vi "desaccade operation.vi"(0 "Data not diff":dbl[][](array[numeric]), 7 "Parameter":T1={"Threshold 1 [Acc]"=0.0, "Threshold 2 [% of TH1]"=0, "tolerance"=2.0, "Search WD "=0.05757575757575758, " always use TH2"=TRUE, "SD for Outliers"=3.0303030303030303, "Max time [ms]"=50.0, "Min time [ms]"=1.0, "Velocity Threshold"=0.05757575757575758} {"Velocity Threshold" scale=50.0..400.0; "SD for Outliers" scale=0.0..5.0; "Search WD" scale=0.0..0.3; "tolerance" scale=0.0..100.0; "Threshold 2 [% of TH1]" scale=0.0..100.0; "Threshold 1 [Acc]" scale=1.0..40000.0}, 11 "Sample Rate":dbl=500.0 format="%.2f") -> (4 "Desaccaded":dbl[][](graph))   [LabVIEW 2016, in "Desaccade Manipulator.lvclass"]
uses:
  Desaccade Manipulator.lvclass
  Typedef - Desaccading Parameter.ctl
  <vilib>/Analysis/3filter.llb/Savitzky-Golay Filter (DBL).vi
  <vilib>/Analysis/NI_AALPro.lvlib
  <vilib>/Analysis/NI_AALBase.lvlib
  comm/nan operations/nan operations.lvlib
panel:
  out "Desaccaded 4":dbl[](graph)
  out "Saccades":dbl[][](graph)
  out "Data Diff & Quadr - Unsmoothed":dbl[][](graph)
  out "Data DIff & Quadr - Smoothed":dbl[][](graph)
  out "Data not differentiated":dbl[][](graph)
  # "Data Input"
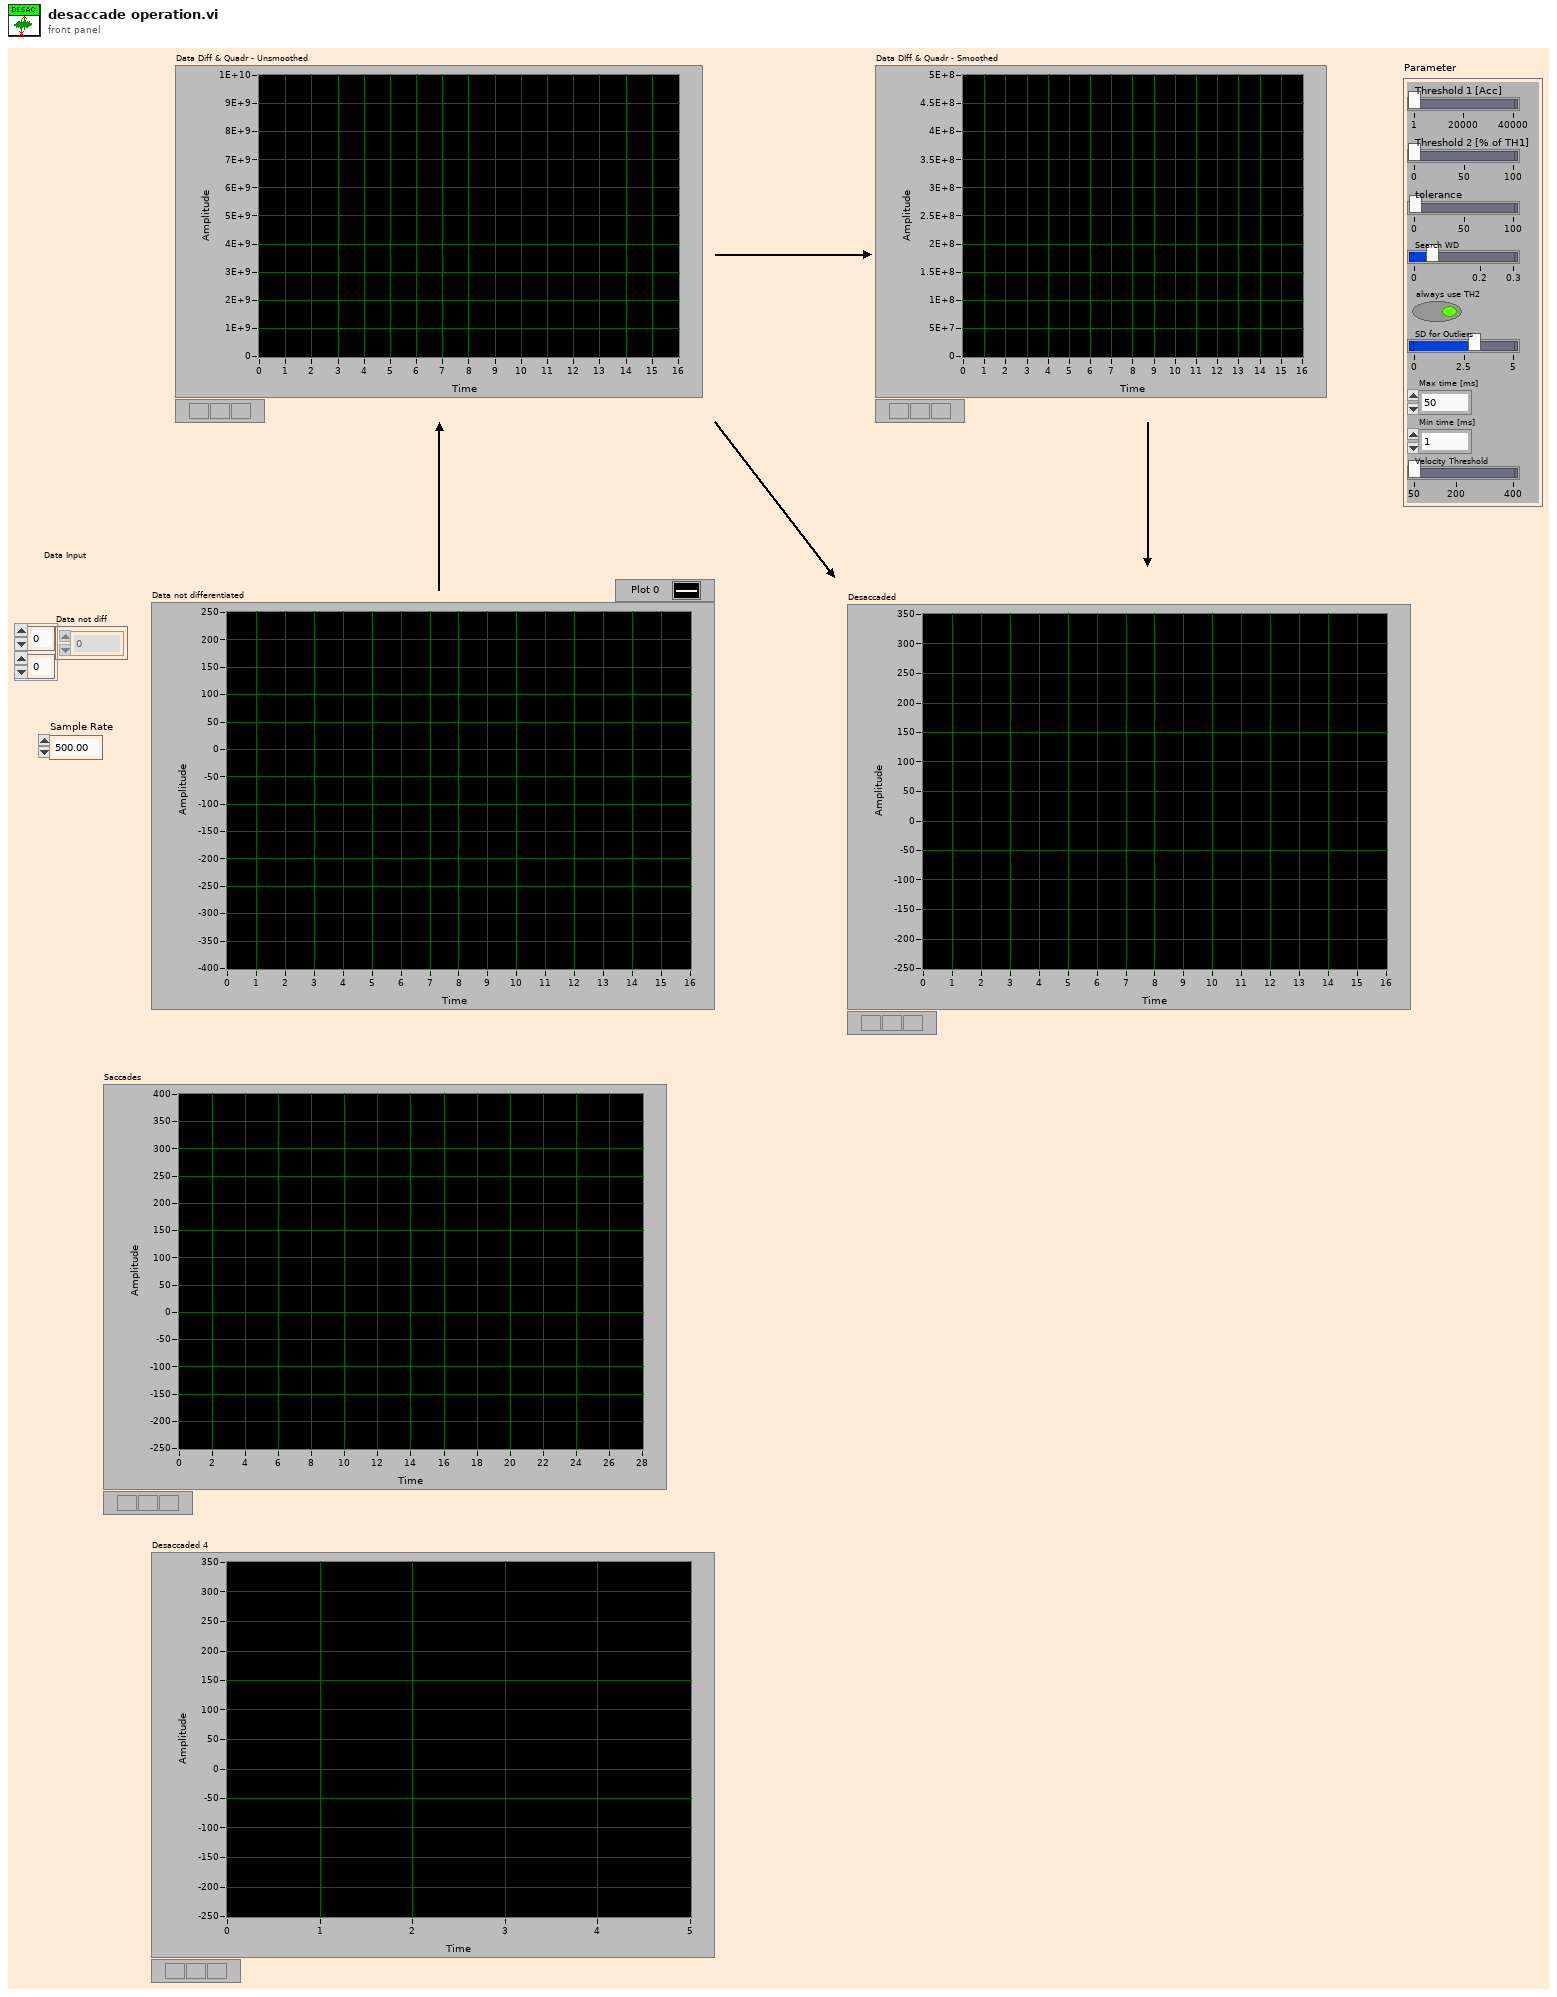
[diagram p1: front panel]
types:
  T1 = typedef "Typedef - Desaccading Parameter.ctl" = cluster{"Threshold 1 [Acc]":dbl, "Threshold 2 [% of TH1]":i32, "tolerance":dbl, "Search WD ":dbl, " always use TH2":bool, "SD for Outliers":dbl, "Max time [ms]":dbl, "Min time [ms]":dbl, "Velocity Threshold":dbl}
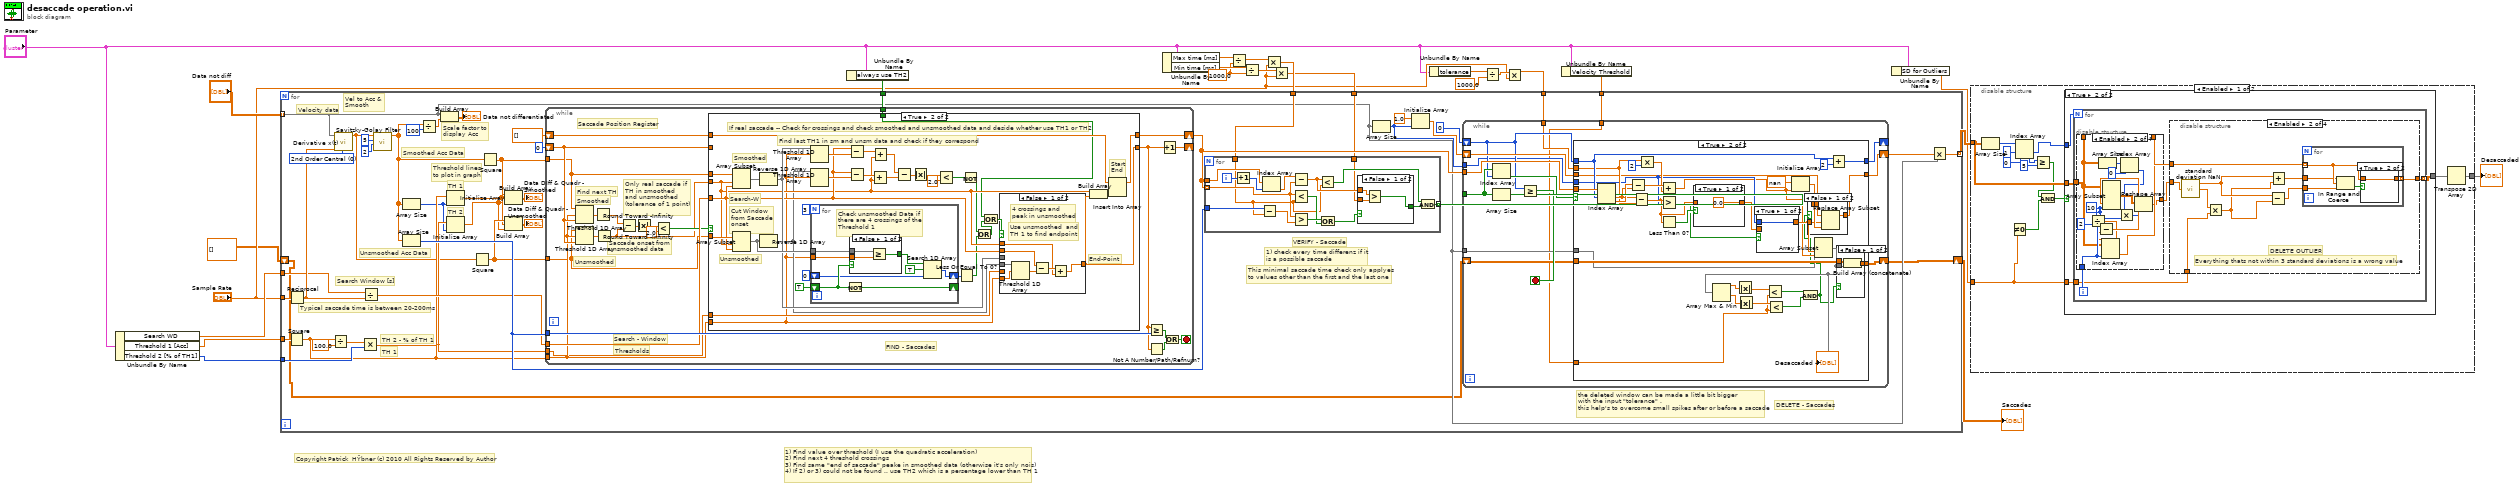
[diagram p0: block diagram]
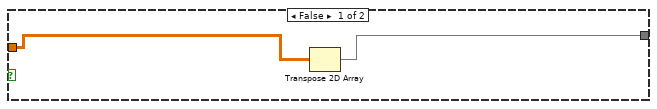
[diagram p2: hidden frame]
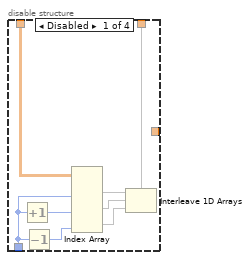
[diagram p3: hidden frame]
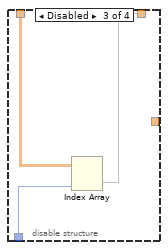
[diagram p4: hidden frame]
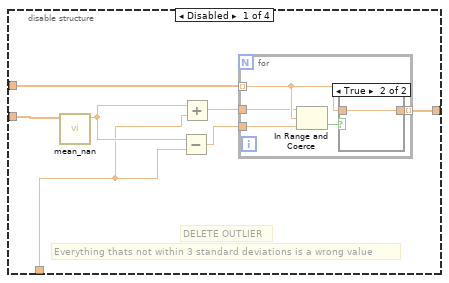
[diagram p6: hidden frame]
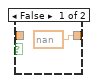
[diagram p7: hidden frame]
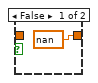
[diagram p8: hidden frame]
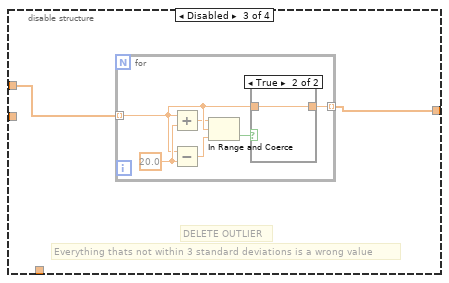
[diagram p9: hidden frame]
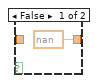
[diagram p10: hidden frame]
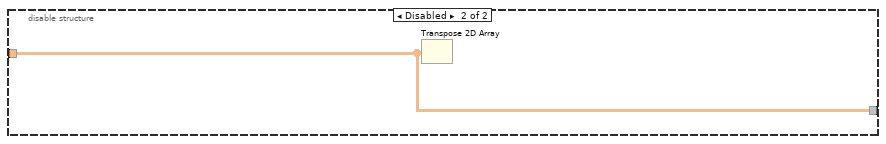
[diagram p12: hidden frame]
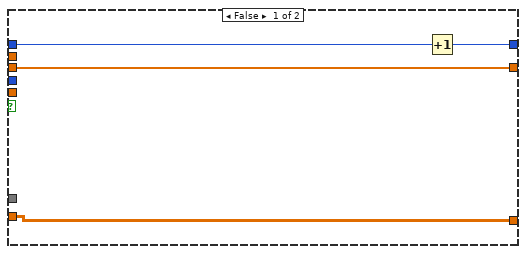
[diagram p13: hidden frame]
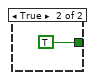
[diagram p18: hidden frame]
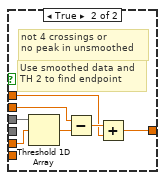
[diagram p20: hidden frame]
diagram:
  w15 = 1000.0 ("y")
  # "1) Find value over threshold (I use the quadratic acceleration)\n2) Find next 4 threshold crossings\n3) Find same \"end of saccade\" peake in smoothed data (otherwise it's only nois)\n4) If 2) or 3) could not be found .. use TH2 which is a persentage lower than TH 1"
  # "Copyright Patrick  HŸbner (c) 2010 All Rights Reserved by Author"
  n1 = Unbundle By Name("Parameter") -> ("Search WD"=w22:dbl, "Threshold 1 [Acc]"=w21:dbl, "Threshold 2 [% of TH1]"=w20:i32)
  n2 = Unbundle By Name("Parameter") -> ("always use TH2"=w19:bool)
  n3 = Unbundle By Name("Parameter") -> ("Max time [ms]"=w17:dbl, "Min time [ms]"=w16:dbl)
  n4 = Divide(x=w17, y=w15) -> (x/y=w14:dbl)
  n5 = Divide(x=w16, y=w15) -> (x/y=w13:dbl)
  n6 = Multiply(x=w14, y="Sample Rate") -> (x*y=w12:dbl)
  n7 = Multiply(x=w13, y="Sample Rate") -> (x*y=w11:dbl)
  n8 = Unbundle By Name("Parameter") -> ("tolerance"=w10:dbl)
  n9 = Divide(x=w10, y=1000.0) -> (x/y=w7:dbl)
  n10 = Multiply(x=w7, y="Sample Rate") -> (x*y=w8:dbl)
  n11 = Unbundle By Name("Parameter") -> ("Velocity Threshold"=w1:dbl)
  n12 = for {
    tunnel: "Sample Rate" -> [w68]
    tunnel: w21 -> [w65]
    tunnel: "Data not diff" -> [w29] mode=indexing
    tunnel: [w35] -> w23 mode=indexing
    tunnel: w20 -> [w51]
    tunnel: w22 -> [w34]
    tunnel: w19 -> [w33]
    tunnel: w12 -> [w32]
    tunnel: w8 -> [w31]
    tunnel: w11 -> [w30]
    shift-right: [w28] -> w3
    shift-left: dbl[][] [] -> [w27]
    tunnel: w1 -> [w26]
    w67 = u16 0 items=["2nd Order Central", "4th Order Central", "Forward", "Backward"] ("method")
    # "DELETE - Saccades"
    # "Scale factor to \ndisplay Acc"
    # "This minimal saccade time check only applyes \nto values other than the first and the last one"
    # "VERIFY - Saccade"
    # "Threshold lines \nto plot in graph"
    # "TH 2"
    # "TH 1"
    # "Vel to Acc &\nSmooth"
    # "Unsmoothed Acc Data"
    # "Smoothed Acc Data"
    # "Velocity data"
    # "Typical saccade time is between 20-200ms"
    # "Search Window [s]"
    # "TH 1"
    # "TH 2 - % of TH 1"
    # "the deleted window can be made a little bit bigger \nwith the input \"tolerance\" . \nthis help's to overcome small spikes after or before a saccade"
    # "1) check every time differenz if it \nis a possible saccade"
    n13 = Square(x=w65) -> (x^2=w47:dbl)
    n14 = Reciprocal(x=w68) -> (1/x=w38:dbl)
    n15 = Divide(x=w47, y=100.0) -> (x/y=w52:dbl)
    n16 = call <vilib>:"Derivative x(t).vi"("method"=w67, "dt"=w38, "X"=w29) -> ("dX/dt"=w25:dbl[])  [unwired: 7 in, 1 out]
    n17 = Multiply(x=w52, y=w51) -> (x*y=w46:dbl)
    n18 = Divide(x=w34, y=w38) -> (x/y=w48:dbl)
    n19 = call-poly <vilib>:"Savitzky-Golay Filter.vi"("polynomial order"=2, "side points"=5, "X"=w25) -> ("Filtered X"=w37:dbl[])  [unwired: 7 in, 1 out]
    n20 = Array Size(array=w37) -> (size(s)=w45:i32)
    n21 = Array Size(array=w37) -> (size(s)=w58:i32)
    n22 = Divide(x=w37, y=100 ("Numeric")) -> (x/y=w55:dbl[])
    n23 = Build Array(w29, w55) -> (→"Data not differentiated":dbl[][])
    n24 = Initialize Array(w47, w45) -> (w40:dbl[])
    n25 = Initialize Array(w46, w45) -> (w39:dbl[])
    n26 = Square(x=w25) -> (x^2=w42:dbl[])
    n27 = Square(x=w37) -> (x^2=w41:dbl[])
    n28 = Build Array(w41, w40, w39) -> (→"Data DIff & Quadr - Smoothed":dbl[][])
    n29 = Build Array(w42, w40, w39) -> (→"Data Diff & Quadr - Unsmoothed":dbl[][])
    n30 = while {
      tunnel: w41 -> [w160]
      shift-right: [w174] -> _
      shift-left: 0 -> [w163]
      shift-right: [w175] -> w60
      shift-left: dbl[] [] ("Filtered X") -> [w173]
      tunnel: w58 -> [w168]
      tunnel: w42 -> [w159]
      tunnel: w48 -> [w165]
      tunnel: w46 -> [w161]
      tunnel: w47 -> [w162]
      tunnel: w33 -> [w154]
      stop <- w167 stop-if-true
      # "FIND - Saccades"
      # "Saccade Position Register"
      # "Only real saccade if\nTH in smoothed\nand unsmoothed \n(tolerance of 1 point)"
      # "Unsmoothed"
      # "Smoothed"
      # "Saccade onset from\nunsmoothed data"
      # "Search - Window"
      # "Thresholds"
      # "Find next TH"
      n31 = Threshold 1D Array(1:w163, 2:w162, 3:w160) -> (0:w176:dbl)
      n32 = Threshold 1D Array(1:w163, 2:w162, 3:w159) -> (0:w172:dbl)
      n33 = Round Toward -Infinity(1:w176) -> (0:w158:dbl)
      n34 = Round Toward -Infinity(1:w172) -> (0:w157:dbl)
      n35 = Subtract(x=w158, y=w157) -> (x-y=w171:dbl)
      n36 = Absolute Value(x=w171) -> (abs(x)=w170:dbl)
      n37 = Less?(x=w170, y=2.0) -> (x < y?=w164:bool)
      n38 = case shown="True" w164 {
        tunnel: [w177 w211] -> w175
        tunnel: w173 -> [w177 w210]
        tunnel: w159 -> [_ w202]
        tunnel: w160 -> [_ w201]
        tunnel: w161 -> [_ w190]
        tunnel: [w178 w189] -> w166
        tunnel: w165 -> [_ w188]
        tunnel: w157 -> [_ w187]
        tunnel: w162 -> [_ w185]
        tunnel: w163 -> [w178 _]
        tunnel: w154 -> [_ w179]
        frame False {
          # "If no real saccade -- Do nothing"
        }
        frame True {
          # "End-Point"
          # "If real saccade -- Check for crossings and check smoothed and unsmoothed data and deside whether use TH1 or TH2"
          # "Find last TH1 in sm and unsm data and check if they correspond"
          # "Smoothed"
          # "Unsmoothed"
          # "Cut Window \nfrom Saccade\nonset"
          # "Search-W"
          # "Start\nEnd"
          n39 = Array Subset(array=w201, index=w187, length=w188) -> (w200:dbl[])
          n40 = Array Subset(array=w202, index=w187, length=w188) -> (w206:dbl[])
          n41 = Reverse 1D Array(array=w200) -> (reversed array=w191:dbl[])
          n42 = Reverse 1D Array(array=w206) -> (reversed array=w186:dbl[])
          n43 = Threshold 1D Array(2:w185, 3:w191) -> (0:w192:dbl)  [unwired: 1 in]
          n44 = Threshold 1D Array(2:w185, 3:w186) -> (0:w199:dbl)  [unwired: 1 in]
          n45 = for {
            N: 3 -> [_]
            tunnel: w206 -> [w233]
            shift-right: [w228] -> _
            shift-left: TRUE -> [w227]
            tunnel: w185 -> [w232]
            shift-right: [w229] -> w203
            shift-left: 0 ("index of element") -> [w226]
            # "Check unsmoothed Data if \nthere are 4 crossings of the \nThreshold 1"
            n46 = Not(x=w227) -> (.not. x?=w228:bool)
            n47 = case shown="False" w227 {
              tunnel: w233 -> [w236 w239]
              tunnel: w232 -> [w235 w238]
              tunnel: [w234 w237] -> w231
              frame False {
                n48 = Greater Or Equal?(x=w236, y=w235) -> (x >= y?=w234:bool[])
              }
              frame True {
                n49 = Less?(x=w239, y=w238) -> (x < y?=w237:bool[])
              }
            }
            n50 = Search 1D Array(1D array=w231, element=TRUE, start index (0)=w226) -> (index of element=w229:i32)
          }
          n51 = Subtract(x=w188, y=w192) -> (x-y=w198:dbl)
          n52 = Subtract(x=w188, y=w199) -> (x-y=w208:dbl)
          n53 = Add(x=w208, y=w187) -> (x+y=w193:dbl)
          n54 = Add(x=w198, y=w187) -> (x+y=w194:dbl)
          n55 = Subtract(x=w194, y=w193) -> (x-y=w197:dbl)
          n56 = Absolute Value(x=w197) -> (abs(x)=w196:dbl)
          n57 = Less?(x=w196, y=2.0) -> (x < y?=w184:bool)
          n58 = Less Or Equal To 0?(x=w203) -> (x <= 0?=w183:bool)
          n59 = Not(x=w184) -> (.not. x?=w182:bool)
          n60 = Or(x=w182, y=w183) -> (x .or. y?=w181:bool)
          n61 = Or(x=w179, y=w181) -> (x .or. y?=w180:bool)
          n62 = case shown="False" w180 {
            tunnel: w191 -> [_ w223]
            tunnel: w190 -> [_ w222]
            tunnel: [w216 w221] -> w189
            tunnel: w188 -> [w215 w220]
            tunnel: w187 -> [w214 w219]
            tunnel: w186 -> [w213 _]
            tunnel: w185 -> [w212 _]
            frame False {
              # "Use unsmoothed  and\nTH 1 to find endpoint"
              # "4 crossings and\npeak in unsmoothed"
              n63 = Threshold 1D Array(2:w212, 3:w213) -> (0:w217:dbl)  [unwired: 1 in]
              n64 = Subtract(x=w215, y=w217) -> (x-y=w218:dbl)
              n65 = Add(x=w218, y=w214) -> (x+y=w216:dbl)
            }
            frame True {
              # "Use smoothed data and\nTH 2 to find endpoint"
              # "not 4 crossings or \nno peak in unsmoothed"
              n66 = Threshold 1D Array(2:w222, 3:w223) -> (0:w224:dbl)  [unwired: 1 in]
              n67 = Subtract(x=w220, y=w224) -> (x-y=w225:dbl)
              n68 = Add(x=w225, y=w219) -> (x+y=w221:dbl)
            }
          }
          n69 = Build Array(w187, w189) -> (w209:dbl[])
          n70 = Insert Into Array(array=w210, new element=w209) -> (w211:dbl[])  [unwired: 1 in]
        }
      }
      n71 = Greater Or Equal?(x=w166, y=w168) -> (x >= y?=w156:bool)
      n72 = Not A Number/Path/Refnum?(number/path/refnum=w166) -> (NaN/Path/Refnum?=w155:bool)
      n73 = Increment(x=w166) -> (x+1=w174:dbl)
      n74 = Or(x=w156, y=w155) -> (x .or. y?=w167:bool)
    }
    n75 = for {
      tunnel: w60 -> [w138] mode=indexing
      tunnel: w60 -> [w149]
      tunnel: [w144] -> w63 mode=indexing
      tunnel: w58 -> [w136]
      tunnel: w32 -> [w135]
      tunnel: w30 -> [w134]
      i -> [w142]
      n76 = Increment(x=w142) -> (x+1=w148:i32)
      n77 = Subtract(x=w136, y=w135) -> (x-y=w137:dbl)
      n78 = Index Array(array=w149, index=w148) -> (element=w147:dbl)
      n79 = Subtract(x=w147, y=w138) -> (x-y=w143:dbl)
      n80 = Less?(x=w138, y=w135) -> (x < y?=w139:bool)
      n81 = Greater?(x=w138, y=w137) -> (0:w141:bool)
      n82 = Less?(x=w143, y=w135) -> (x < y?=w146:bool)
      n83 = Or(x=w141, y=w139) -> (x .or. y?=w140:bool)
      n84 = case shown="False" w140 {
        tunnel: w134 -> [w152 _]
        tunnel: [w151 TRUE] -> w145
        tunnel: w143 -> [w150 _]
        frame False {
          n85 = Greater?(x=w150, y=w152) -> (0:w151:bool)
        }
        frame True {
        }
      }
      n86 = And(x=w146, y=w145) -> (x .and. y?=w144:bool)
    }
    n87 = Array Size(array=w29) -> (size(s)=w57:i32)
    n88 = Initialize Array(1.0 ("element"), w57) -> (w61:dbl[])
    n89 = while {
      tunnel: w60 -> [w82]
      shift-right: [w80] -> w36
      shift-left: w61 -> [w81]
      shift-right: [w78] -> _
      shift-left: 0 -> [w75]
      tunnel: w63 -> [w79]
      tunnel: w57 -> [w74]
      tunnel: w31 -> [w73]
      shift-right: [w72] -> w28
      shift-left: w27 -> [w71]
      tunnel: w29 -> [w70]
      tunnel: w26 -> [w69]
      stop <- w77 stop-if-true
      n90 = Index Array(array=w79, index=w75) -> (element=w83:bool)
      n91 = Array Size(array=w79) -> (size(s)=w76:i32)
      n92 = Greater Or Equal?(x=w75, y=w76) -> (x >= y?=w77:bool)
      n93 = case shown="True" w83 {
        tunnel: w82 -> [_ w120]
        tunnel: w81 -> [w87 w99]
        tunnel: [w87 w115] -> w80
        tunnel: w75 -> [w86 w113]
        tunnel: [w85 w114] -> w78
        tunnel: w73 -> [_ w108]
        tunnel: w74 -> [_ w103]
        tunnel: [w84 w102] -> w72
        tunnel: w71 -> [w84 w101]
        tunnel: w70 -> [_ w100]
        tunnel: w69 -> [_ w88]
        frame False {
          n94 = Increment(x=w86) -> (x+1=w85:i32)
        }
        frame True {
          n95 = Index Array(array=w120, index #1=w113) -> (element #1=w109:dbl, element #2=w119:dbl)  [unwired: 1 in]
          n96 = Subtract(x=w119, y=w109) -> (x-y=w117:dbl)
          n97 = Subtract(x=w109, y=w108) -> (x-y=w106:dbl)
          n98 = Multiply(x=w108, y=2) -> (x*y=w110:dbl)
          n99 = Add(x=w117, y=w110) -> (x+y=w97:dbl)
          n100 = Greater?(x=w106, y=w103) -> (0:w105:bool)
          n101 = Less Than 0?(x=w106) -> (x < 0?=w107:bool)
          n102 = case shown="True" w107 {
            tunnel: w106 -> [_ w133]
            tunnel: [0.0 w133] -> w104
            frame True {
            }
            frame False {
            }
          }
          n103 = case shown="True" w105 {
            tunnel: w104 -> [_ w131]
            tunnel: [w130 w131] -> w98
            tunnel: w103 -> [w130 _]
            frame True {
            }
            frame False {
            }
          }
          n104 = Initialize Array(nan, w97) -> (w116:dbl[])
          n105 = Array Subset(array=w100, index=w98, length=w97) -> (w90:dbl[])
          "Desaccaded 4" <- w90
          n106 = Array Max & Min(array=w90) -> (max value=w96:dbl, min value=w95:dbl)  [unwired: 2 out]
          n107 = Absolute Value(x=w96) -> (abs(x)=w94:dbl)
          n108 = Absolute Value(x=w95) -> (abs(x)=w93:dbl)
          n109 = Less?(x=w94, y=w88) -> (x < y?=w92:bool)
          n110 = Less?(x=w93, y=w88) -> (x < y?=w91:bool)
          n111 = And(x=w92, y=w91) -> (x .and. y?=w89:bool)
          n112 = case shown="False" w89 {
            tunnel: w116 -> [w128 _]
            tunnel: [w127 w129] -> w115
            tunnel: w99 -> [w126 w129]
            tunnel: w98 -> [w125 _]
            frame False {
              n113 = Replace Array Subset(array=w126, new element=w128, index=w125) -> (w127:dbl[])
            }
            frame True {
            }
          }
          n114 = Add(x=w113, y=2) -> (x+y=w114:i32)
          n115 = case shown="False" w89 {
            tunnel: [w123 w124] -> w102
            tunnel: w101 -> [w122 w124]
            tunnel: w90 -> [w121 _]
            frame False {
              n116 = Build Array (concatenate)(w122, w121) -> (w123:dbl[][])
            }
            frame True {
            }
          }
        }
      }
    }
    n117 = Multiply(x=w36, y=w29) -> (x*y=w35:dbl[])
  }
  "Saccades" <- w3
  n118 = Unbundle By Name("Parameter") -> ("SD for Outliers"=w18:dbl)
  n119 = disable-structure shown="Enabled" {
    disable-tunnel: [w249 w328] -> w4
    disable-tunnel: w23 -> [w248 w328]
    disable-tunnel: w18 -> [w240 _]
    frame Enabled {
      n120 = Array Size(array=w248) -> (size(s)=w252:i32[])
      n121 = Not Equal To 0?(x=w240) -> (x != 0?=w241:bool)
      n122 = Index Array(array=w252, index #1=1 ("index"), index #2=0 ("index")) -> (element #1=w247:i32, element #2=w245:i32)
      n123 = Greater Or Equal?(x=w245, y=5) -> (x >= y?=w242:bool)
      n124 = And(x=w242, y=w241) -> (x .and. y?=w243:bool)
      n125 = case shown="True" w243 {
        tunnel: [w253 w258] -> w250
        tunnel: w248 -> [w254 w257]
        tunnel: w247 -> [_ w256]
        tunnel: w240 -> [_ w255]
        frame False {
          n126 = Transpose 2D Array(2D array=w254) -> (transposed array=w253:dbl[][])
        }
        frame True {
          n127 = for {
            N: w256 -> [_]
            tunnel: w257 -> [w263]
            tunnel: [w264] -> w258 mode=indexing
            tunnel: w255 -> [w260]
            i -> [w261]
            n128 = disable-structure shown="Enabled" {
              disable-tunnel: w263 -> [w271 w277 w287 _]
              disable-tunnel: [w267 w284 w285 _] -> w262
              disable-tunnel: w261 -> [w265 w281 w286 _]
              disable-tunnel: [_ w279 _ _] -> w259
              frame Disabled {
                n129 = Increment(x=w265) -> (x+1=w270:i32)
                n130 = Decrement(x=w265) -> (x-1=w266:i32)
                n131 = Index Array(array=w271, index (col) #1=w265, index (col) #2=w270, index (col) #3=w266) -> (element #1=w267:dbl[], element #2=w269:dbl[], element #3=w268:dbl[])  [unwired: 3 in]
                n132 = Interleave 1D Arrays(w267, w269, w268) -> ()  [unwired: 1 out]
              }
              frame Enabled {
                w275 = 10 ("length")
                n133 = Divide(x=w275, y=2) -> (x/y=w280:dbl)
                n134 = Subtract(x=w281, y=w280) -> (x-y=w283:dbl)
                n135 = Array Size(array=w277) -> (size(s)=w274:i32[])
                n136 = Index Array(array=w277, index (col)=w281) -> (element=w284:dbl[])  [unwired: 1 in]
                n137 = Array Subset(array=w277, index (col)=w283, length (col)=w275) -> (w278:dbl[][])  [unwired: 2 in]
                n138 = Index Array(array=w274, index=0) -> (element=w273:i32)
                n139 = Multiply(x=w273, y=w275) -> (x*y=w272:i32)
                n140 = Reshape Array(w278, w272) -> (w279:dbl[])
              }
              frame Disabled {
                n141 = Index Array(array=w287, index (col)=w286) -> (element=w285:dbl[])  [unwired: 1 in]
              }
              frame Disabled {
              }
            }
            n142 = disable-structure shown="Enabled" {
              disable-tunnel: [w294 w310 w319 _] -> w264
              disable-tunnel: w259 -> [w293 w309 _ _]
              disable-tunnel: w262 -> [w292 w308 w318 _]
              disable-tunnel: w260 -> [w288 w303 _ _]
              frame Disabled {
                # "DELETE OUTLIER"
                # "Everything thats not within 3 standard deviations is a wrong value"
                n143 = call "mean_nan.vi"("Array"=w293) -> ("Mean"=w291:dbl)  [unwired: 10 in]
                n144 = Subtract(x=w291, y=w288) -> (x-y=w290:dbl)
                n145 = Add(x=w291, y=w288) -> (x+y=w289:dbl)
                n146 = for {
                  tunnel: [w298] -> w294 mode=indexing
                  tunnel: w292 -> [w297] mode=indexing
                  tunnel: w290 -> [w296]
                  tunnel: w289 -> [w295]
                  n147 = In Range and Coerce(upper limit=w295, x=w297, lower limit=w296) -> (In Range?=w299:bool)  [unwired: 1 out]
                  n148 = case shown="True" w299 {
                    tunnel: [nan w301] -> w298
                    tunnel: w297 -> [_ w301]
                    frame False {
                    }
                    frame True {
                    }
                  }
                }
              }
              frame Enabled {
                # "DELETE OUTLIER"
                # "Everything thats not within 3 standard deviations is a wrong value"
                n149 = call "standard deviation NaN.vi"("Array"=w309) -> ("standard deviation"=w304:dbl, "mean"=w307:dbl)  [unwired: 2 in, 1 out]
                n150 = Multiply(x=w304, y=w303) -> (x*y=w302:dbl)
                n151 = Subtract(x=w307, y=w302) -> (x-y=w306:dbl)
                n152 = Add(x=w307, y=w302) -> (x+y=w305:dbl)
                n153 = for {
                  tunnel: [w314] -> w310 mode=indexing
                  tunnel: w308 -> [w313] mode=indexing
                  tunnel: w306 -> [w312]
                  tunnel: w305 -> [w311]
                  n154 = In Range and Coerce(upper limit=w311, x=w313, lower limit=w312) -> (In Range?=w315:bool)  [unwired: 1 out]
                  n155 = case shown="True" w315 {
                    tunnel: [nan w317] -> w314
                    tunnel: w313 -> [_ w317]
                    frame False {
                    }
                    frame True {
                    }
                  }
                }
              }
              frame Disabled {
                # "DELETE OUTLIER"
                # "Everything thats not within 3 standard deviations is a wrong value"
                n156 = for {
                  tunnel: [w324] -> w319 mode=indexing
                  tunnel: w318 -> [w322] mode=indexing
                  w323 = 20.0 ("y")
                  n157 = Add(x=w322, y=w323) -> (x+y=w320:dbl)
                  n158 = Subtract(x=w322, y=w323) -> (x-y=w321:dbl)
                  n159 = In Range and Coerce(upper limit=w320, x=w322, lower limit=w321) -> (In Range?=w325:bool)  [unwired: 1 out]
                  n160 = case shown="True" w325 {
                    tunnel: [nan w327] -> w324
                    tunnel: w322 -> [_ w327]
                    frame False {
                    }
                    frame True {
                    }
                  }
                }
              }
              frame Disabled {
              }
            }
          }
        }
      }
      n161 = Transpose 2D Array(2D array=w250) -> (transposed array=w249:dbl[][])
    }
    frame Disabled {
      n162 = Transpose 2D Array(2D array=w328) -> (transposed array=w329:dbl[][])
    }
  }
  "Desaccaded" <- w4
